vi "AM_Tx_Template.vi"() -> ()   [LabVIEW 2018]
uses:
  <instrlib>/niUSRP/niUSRP Write Tx Data (CDB).vi
  <vilib>/measure/NI_MAPro.lvlib
panel:
  out "Baseband Signal":dbl[](graph)
  out "Message Signal":waveform(dbl)(graph)
  out "Error out":errorcluster
  in  "stop":bool
  in  "Modulation Index":dbl=1.0 min=0.0 max=1.0
  in  "# Tones":i32=3
  in  "Delta Frequency":dbl=1000.0 format="%.2p"
  in  "Start Frequency":dbl=1000.0 format="%.2p"
  in  "Message Length\n(samples)":dbl=200000.0
  in  "Active Antenna":string(combo)="TX1"
  out "Actual Gain (dB)":dbl format="%#_6f"
  in  "Gain (dB)":dbl=20.0 min=0.0 max=31.0 format="%#_6f"
  out "Actual Frequency":dbl=100000.0 format="%#_6p"
  in  "Carrier Frequency":dbl=915100000.0 format="%#_6p"
  out "Actual IQ Rate":dbl=100000.0 format="%#_6p"
  in  "IQ Rate":dbl=200000.0 format="%#_6p"
  in  "Device Names":refnum<k15>="192.168.10.2"
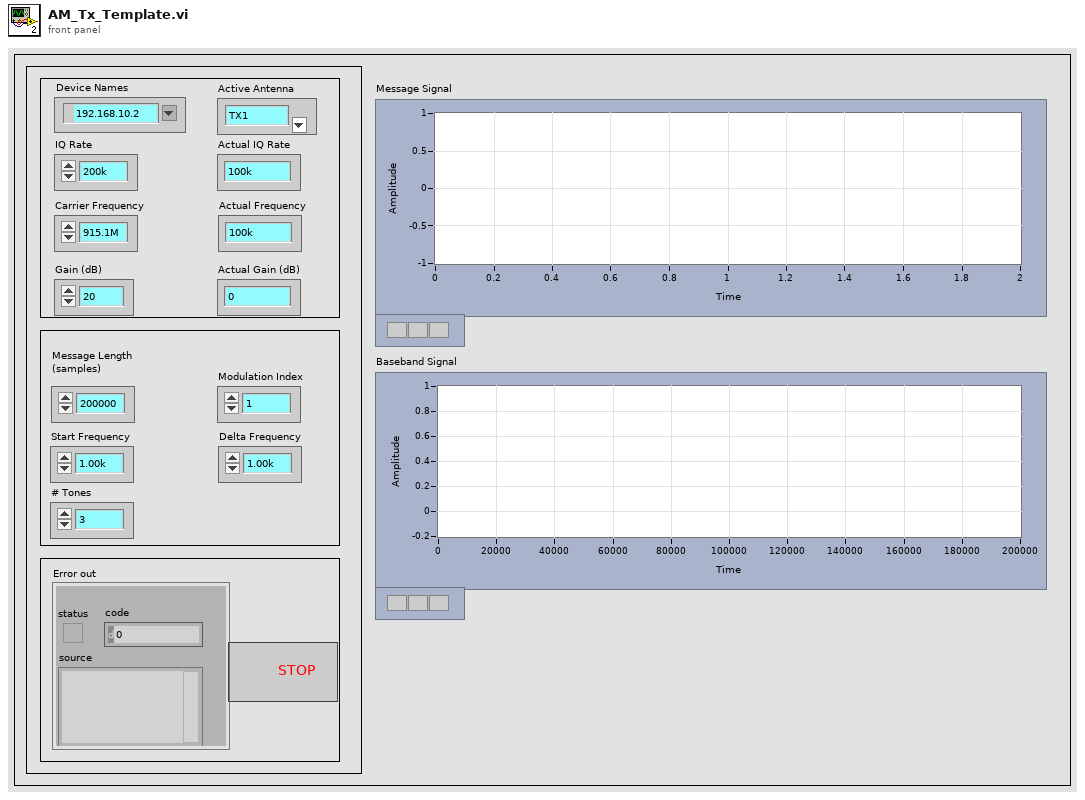
[diagram p1: front panel]
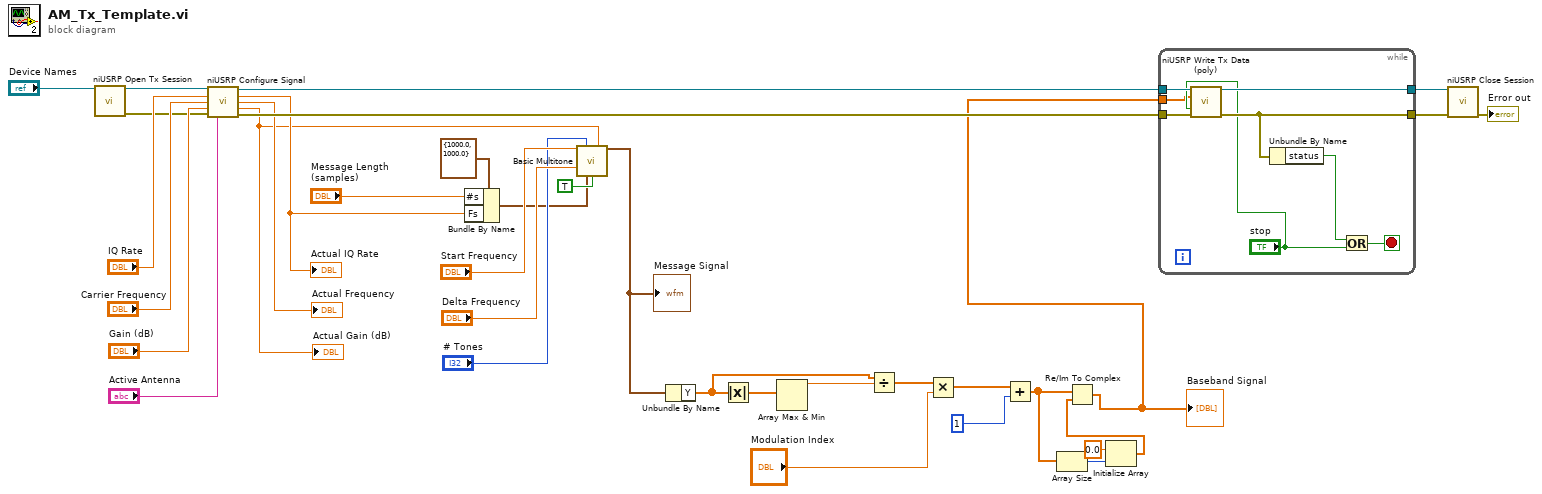
[diagram p0: block diagram]
diagram:
  n1 = call <instrlib>:"niUSRP Open Tx Session.vi"("device names"="Device Names") -> ("session handle out"=w34:refnum<k15>, "error out"=w30:errorcluster)  [unwired: 13 in]
  n2 = call <instrlib>:"niUSRP Configure Signal.vi"("session handle"=w34, "IQ rate"="IQ Rate", "carrier frequency"="Carrier Frequency", "gain"="Gain (dB)", "error in (no error)"=w30, "active antenna"="Active Antenna") -> ("session handle out"=w24:refnum<k15>, "coerced IQ rate"=w16:dbl, "coerced carrier frequency"=→"Actual Frequency":dbl, "coerced gain"=w14:dbl, "error out"=w22:errorcluster)  [unwired: 5 in]
  "Actual IQ Rate" <- w16
  "Actual Gain (dB)" <- w14
  n3 = Bundle By Name(cluster=cluster{"Fs":dbl, "#s":dbl} {"Fs"=1000.0, "#s"=1000.0} ("sampling info"), "#s"="Message Length\n(samples)", "Fs"=w16) -> (w17:cluster{"Fs":dbl, "#s":dbl})
  n4 = call <vilib>:"Basic Multitone.vi"("start frequency"="Start Frequency", "#tones"="# Tones", "amplitude"=w14, "delta frequency"="Delta Frequency", "sampling info"=w17, "coerce frequencies?"=TRUE) -> ("signal out"=w13:waveform(dbl))  [unwired: 6 in, 3 out]
  "Message Signal" <- w13
  n5 = Unbundle By Name(w13) -> ("Y"=w10:dbl[])
  n6 = Absolute Value(x=w10) -> (abs(x)=w12:dbl[])
  n7 = Array Max & Min(array=w12) -> (max value=w11:dbl)  [unwired: 3 out]
  n8 = Divide(x=w10, y=w11) -> (x/y=w9:dbl[])
  n9 = Multiply(x=w9, y="Modulation Index") -> (x*y=w7:dbl[])
  n10 = Add(x=w7, y=1) -> (x+y=w4:dbl[])
  n11 = Array Size(array=w4) -> (size(s)=w3:i32)
  n12 = Initialize Array(0.0 ("element"), w3) -> (w1:dbl[])
  n13 = Re/Im To Complex(1:w1, 2:w4) -> (0:w5:cdb[])
  "Baseband Signal" <- w5
  n14 = while {
    tunnel: w24 -> [w43]
    tunnel: [w42] -> w23
    tunnel: w22 -> [w41]
    tunnel: [w40] -> w19
    tunnel: w5 -> [w36]
    stop <- w38 stop-if-true
    n15 = call-poly <instrlib>:"niUSRP Write Tx Data (poly).vi"("session handle"=w43, "data"=w36, "end of data?"="stop", "error in (no error)"=w41) -> ("session handle out"=w42:refnum<k15>, "error out"=w40:errorcluster)  [unwired: 10 in]
    n16 = Unbundle By Name(w40) -> ("status"=w39:bool)
    n17 = Or(x=w39, y="stop") -> (x .or. y?=w38:bool)
  }
  n18 = call <instrlib>:"niUSRP Close Session.vi"("session handle"=w23, "error in (no error)"=w19) -> ("error out"=→"Error out":errorcluster)  [unwired: 13 in]
